vi "Get_Laser_Status.vi"(8 "error in (no error)":errorcluster, 11 "connection ID":refnum<k5>) -> (0 "error out":errorcluster, 1 "Checksum OK":bool, 2 "init_cluster":T1, 3 "connection ID out":refnum<k5>)   [LabVIEW 2021]
uses:
  TypeDefs/laser_cabinet_status.ctl
panel:
  out "Answer":u16
  out "Execution code`":u16
  out "Data size":u32
  out "length":i32
  out "data in":string
  out "Data":string
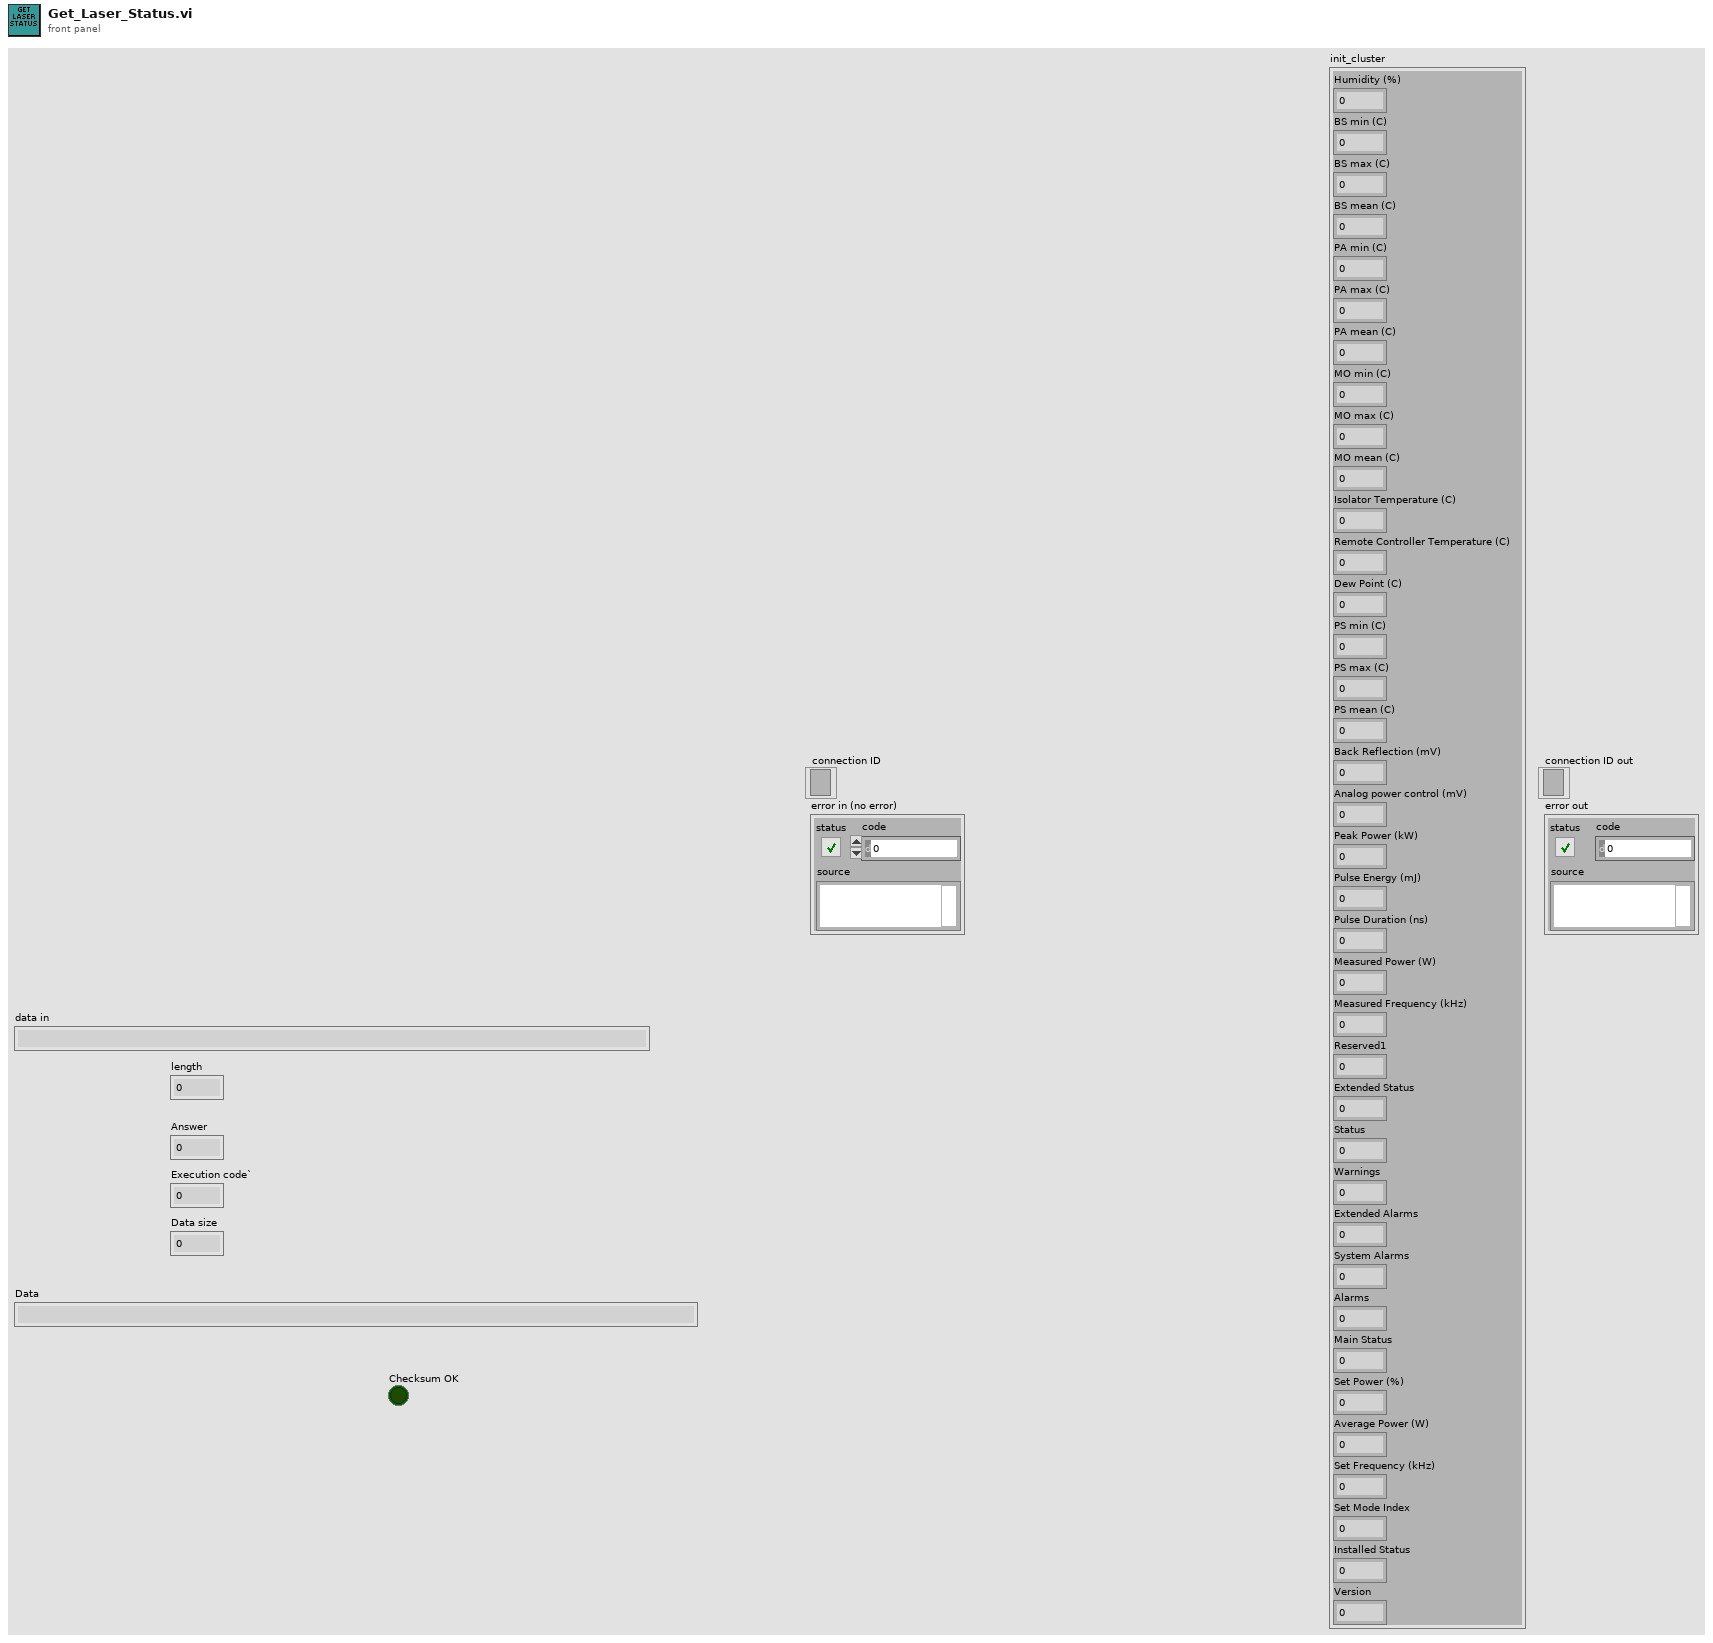
[diagram p1: front panel]
types:
  T1 = typedef "laser_cabinet_status.ctl" = cluster{"Version":u16, "Installed Status":u32, "Set Mode Index":u16, "Set Frequency (kHz)":sgl, "Average Power (W)":sgl, "Set Power (%)":sgl, "Main Status":u32, "Alarms":u32, "System Alarms":u32, "Extended Alarms":u32, "Warnings":u32, "Status":u32, "Extended Status":u32, "Reserved1":u16, "Measured Frequency (kHz)":sgl, "Pulse Duration (ns)":u32, "Measured Power (W)":sgl, "Pulse Energy (mJ)":sgl, "Peak Power (kW)":sgl, "Analog power control (mV)":sgl, "Back Reflection (mV)":sgl, "PS mean (C)":sgl, "PS max (C)":sgl, "PS min (C)":sgl, "Dew Point (C)":sgl, "Remote Controller Temperature (C)":sgl, "Isolator Temperature (C)":sgl, "MO mean (C)":sgl, "MO max (C)":sgl, "MO min (C)":sgl, "PA mean (C)":sgl, "PA max (C)":sgl, "PA min (C)":sgl, "BS mean (C)":sgl, "BS max (C)":sgl, "BS min (C)":sgl, "Humidity (%)":sgl}
  T2 = enum16{"big-endian, network order", "native, host order", "little-endian"}
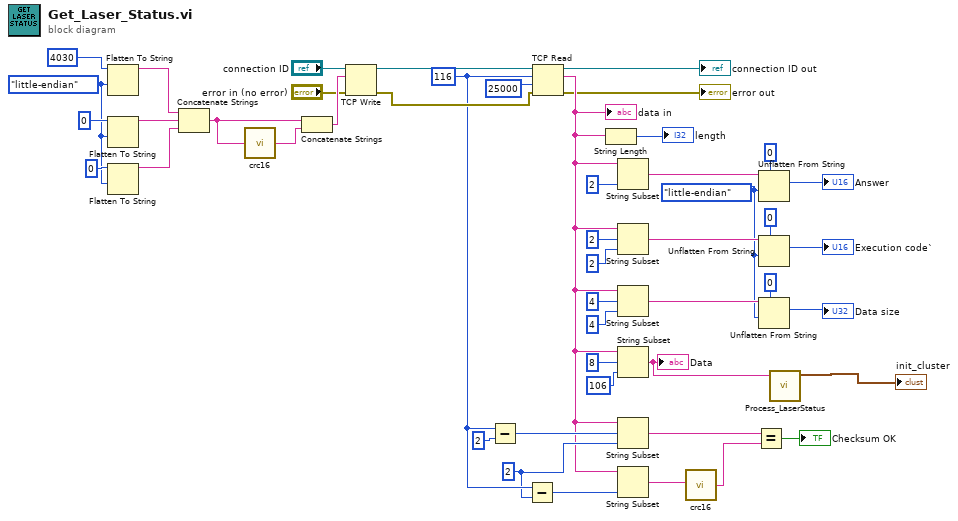
[diagram p0: block diagram]
diagram:
  w13 = T2."little-endian" ("byte order (0:big-endian, network order)")
  w21 = T2."little-endian" ("byte order (0:big-endian, network order)")
  w33 = 2 ("length (rest)")
  w34 = 116 ("bytes to read")
  n1 = Flatten To String(anything=u16 4030 ("Command"), byte order (0:big-endian, network order)=w21) -> (data string=w28:string)  [unwired: 2 in, 2 out]
  n2 = Flatten To String(anything=u16 0, byte order (0:big-endian, network order)=w21) -> (data string=w27:string)  [unwired: 2 in, 2 out]
  n3 = Flatten To String(anything=u32 0 ("Datasize"), byte order (0:big-endian, network order)=w21) -> (data string=w26:string)  [unwired: 2 in, 2 out]
  n4 = Concatenate Strings(w28, w27, w26) -> (w8:string)
  n5 = call "crc16.vi"("string"=w8) -> ("string 2"=w9:string)
  n6 = Concatenate Strings(w8, w9) -> (w42:string)
  n7 = TCP Write(connection ID="connection ID", data in=w42, error in (no error)="error in (no error)") -> (connection ID out=w47:refnum<k5>, error out=w45:errorcluster)  [unwired: 1 in, 1 out]
  n8 = Subtract(x=w34, y=2 ("offset (0)")) -> (x-y=w36:i32)
  n9 = Subtract(x=w34, y=w33) -> (x-y=w32:i32)
  n10 = TCP Read(connection ID=w47, bytes to read=w34, error in (no error)=w45, 9:25000 ("timeout ms (25000)")) -> (connection ID out=→"connection ID out":refnum<k5>, data out=w25:string, error out=→"error out":errorcluster)  [unwired: 1 in]
  "data in" <- w25
  n11 = String Length(string=w25) -> (length=→"length":i32)
  n12 = String Subset(string=w25, length (rest)=2 ("length (rest)")) -> (substring=w19:string)  [unwired: 1 in]
  n13 = String Subset(string=w25, offset (0)=2, length (rest)=2 ("length (rest)")) -> (substring=w17:string)
  n14 = String Subset(string=w25, offset (0)=4, length (rest)=4 ("length (rest)")) -> (substring=w14:string)
  n15 = String Subset(string=w25, offset (0)=8, length (rest)=106 ("length (rest)")) -> (substring=w10:string)
  "Data" <- w10
  n16 = String Subset(string=w25, offset (0)=w36, length (rest)=w33) -> (substring=w35:string)
  n17 = String Subset(string=w25, length (rest)=w32) -> (substring=w7:string)  [unwired: 1 in]
  n18 = call "crc16.vi"("string"=w7) -> ("string 2"=w4:string)
  n19 = Equal?(x=w35, y=w4) -> (x = y?=→"Checksum OK":bool)
  n20 = Unflatten From String(type=u16 0, binary string=w19, byte order (0:big-endian, network order)=w13) -> (value=→"Answer":u16)  [unwired: 2 in, 2 out]
  n21 = Unflatten From String(type=u16 0, binary string=w17, byte order (0:big-endian, network order)=w13) -> (value=→"Execution code`":u16)  [unwired: 2 in, 2 out]
  n22 = Unflatten From String(type=u32 0, binary string=w14, byte order (0:big-endian, network order)=w13) -> (value=→"Data size":u32)  [unwired: 2 in, 2 out]
  n23 = call "Process_LaserStatus.vi"("Data"=w10) -> ("output cluster"=→"init_cluster":T1)  [unwired: 10 in]
